vi "Read-Write Config..vi"(8 "error in":errorcluster, 9 "Enum":enum16{"Write", "Read"}(ring), 10 "file path (use dialog)":path, 11 "Write Data":T1(array[cluster])) -> (0 "error out":errorcluster, 3 "Read Data":T1(array[cluster]))   [LabVIEW 2015]
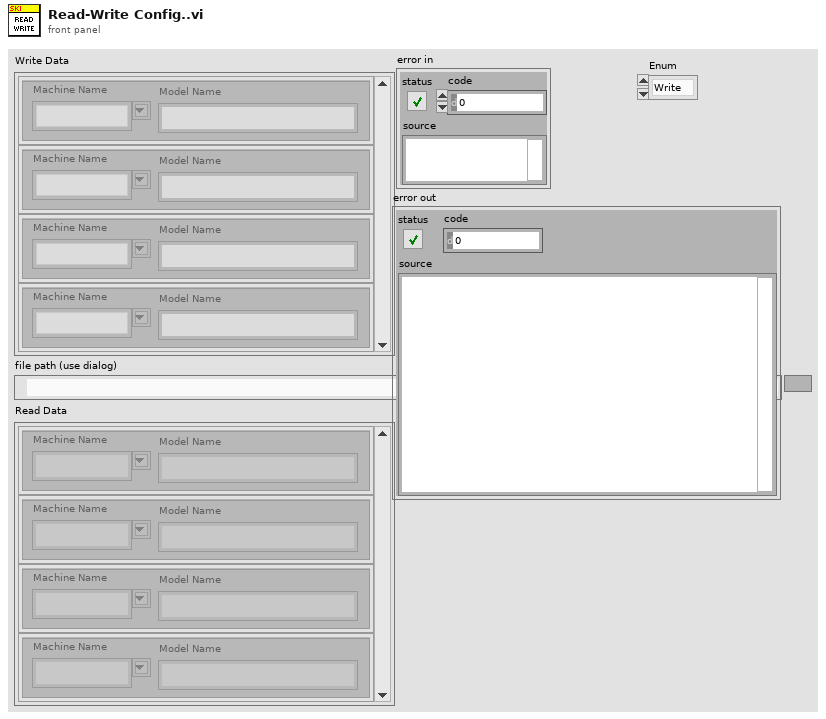
[diagram p1: front panel]
types:
  T1 = cluster{"Machine Name":string, "Model Name":string}[]
  T2 = enum16{"open", "replace", "create", "open or create", "replace or create", "replace or create with confirmation"}
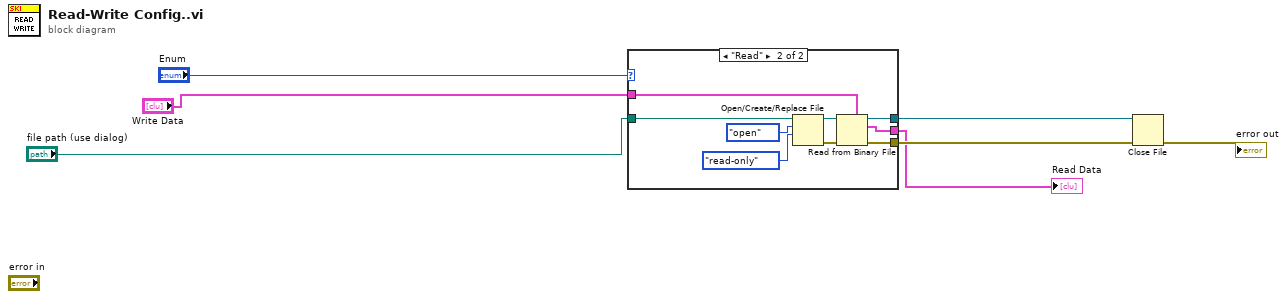
[diagram p0: block diagram]
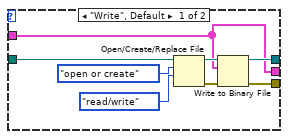
[diagram p2: hidden frame]
diagram:
  n1 = case shown="\"Read\"" "Enum" {
    tunnel: [w15 w23] -> w6
    tunnel: [w14 w24] -> w5
    tunnel: "Write Data" -> [w8 w22]
    tunnel: [w8 w21] -> w4
    tunnel: "file path (use dialog)" -> [w12 w16]
    frame "Write", Default {
      n2 = Open/Create/Replace File(file path (use dialog)=w12, operation (0:open)=T2."open or create", access (0:read/write)=enum16{"read/write", "read-only", "write-only"}."read/write") -> (refnum out=w13:refnum<file>, error out=w9:errorcluster)  [unwired: 3 in, 1 out]
      n3 = Write to Binary File(file (use dialog)=w13, data=w8, error in=w9) -> (refnum out=w15:refnum<file>, error out=w14:errorcluster)  [unwired: 3 in, 1 out]
    }
    frame "Read" {
      n4 = Open/Create/Replace File(file path (use dialog)=w16, operation (0:open)=T2."open", access (0:read/write)=enum16{"read/write", "read-only", "write-only"}."read-only") -> (refnum out=w17:refnum<file>, error out=w18:errorcluster)  [unwired: 3 in, 1 out]
      n5 = Read from Binary File(5:w22, 8:w18, 11:w17) -> (0:w24:errorcluster, 2:w21:T1, 3:w23:refnum<file>)  [unwired: 3 in, 1 out]
    }
  }
  "Read Data" <- w4
  n6 = Close File(refnum=w6, error in=w5) -> (error out=→"error out":errorcluster)  [unwired: 1 out]
